vi "Configure Device.vi"(8 "error in":errorcluster, 11 "Vaisala Probe in":refnum<class "Vaisala.lvclass">) -> (0 "error out":errorcluster, 3 "Vaisala Probe out":refnum<class "Vaisala.lvclass">, 4 "SP":dbl, 5 "Settable?":bool)   [LabVIEW 2014, in "Vaisala Library.lvlib" / "Vaisala.lvclass"]
doc: "Configure the current instance of the Vaisala probe. In this case, we will get the correct address and then set the serial delayso that the probe responds in the correct amount of time. When configuration is done, make sure the session is closed."
uses:
  Vaisala.lvclass
  reusable/Session APIs/Serial/Serial Session.lvclass
  Configurable Device/Configurable Device.lvclass/Configurable Device.ctl
  reusable/Session APIs/File Access/Config Data/Config Data.lvclass/Config Data.ctl
  Vaisala.lvclass/Vaisala.ctl
  Configurable Device/Read ID.vi
  Configurable Device/Read Handle.vi
  Configurable Device/Read Log Session.vi
  Configurable Device/Accessors/Write type.vi
  Configurable Device/Accessors/Write controller_.vi
  reusable/Session APIs/File Access/Config Data/Accessors/Read Ref.vi
  Accessors/Write hSession.vi
  Accessors/Write Address.vi
  Configurable Device/Accessors/Write label.vi
  <vilib>/Utility/config.llb/Read Key (I32).vi
  <vilib>/Utility/config.llb/Read Key (String).vi
  Configurable Device/Configurable Device.lvclass
  reusable/Session APIs/File Access/Config Data/Config Data.lvclass
  <userlib>/_Session Fwk/Session - Root.lvclass
  <vilib>/Utility/config.llb/NI_LVConfig.lvlib
  reusable/Session APIs/Session Log/System Log.lvclass
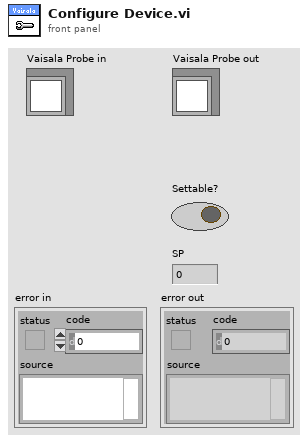
[diagram p1: front panel]
types:
  T1 = typedef "Config Data.lvclass/Config Session.ctl" = refnum<data-value>
  T2 = typedef "Session - Root.lvclass/Session Handle.ctl" = refnum<data-value>
  T3 = typedef "Serial Session.lvclass/Session Handle.ctl" = refnum<data-value>
  T4 = typedef "NI_LVConfig.lvlib/Config Data RefNum.ctl" = refnum<k1>
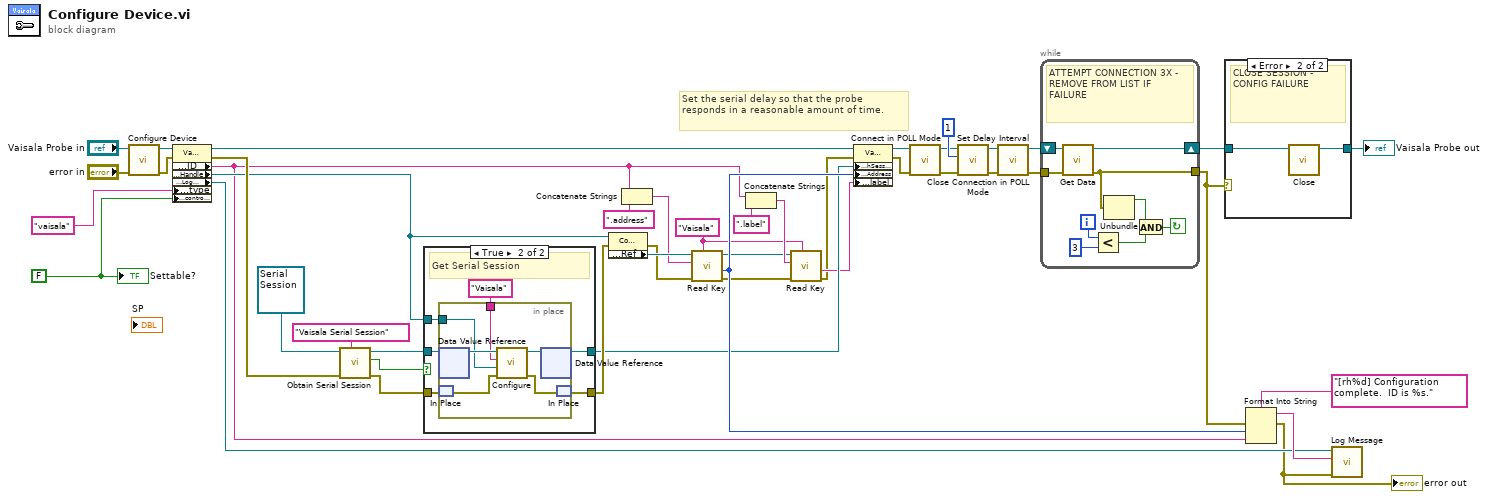
[diagram p0: block diagram]
diagram:
  w14 = FALSE ("controller_")
  w6 = "Vaisala" ("section")
  # "Set the serial delay so that the probe responds in a reasonable amount of time."
  n1 = call-parent "Configure Device.vi"("error in"="error in", "Device in"="Vaisala Probe in") -> ("error out"=w10:errorcluster, "Device out"=w11:refnum<class "Vaisala.lvclass">)  [unwired: 6 in, 2 out]
  n2 = property class="Vaisala"(reference=w11, error in=w10, "Accessors:type"="vaisala" ("type"), "Accessors:controller_"=w14) -> (reference out=w38:refnum<class "Vaisala.lvclass">, error out=w34:errorcluster, "Accessors:ID"=w1:string, "Accessors:Handle"=w31:T1, "Accessors:Log Session"=w32:T2)
  n3 = call "Obtain Serial Session.vi"("Session Name ()"="Vaisala Serial Session", "error in"=w34, "Serial Session in"=refnum<class "Serial Session.lvclass"> refnum) -> ("error out"=w35:errorcluster, "created new?"=w36:bool, "hSerial"=w39:T3)  [unwired: 6 in]
  n4 = case shown="True" w36 {
    tunnel: w39 -> [w47 w53]
    tunnel: w35 -> [w46 w50]
    tunnel: [w47 w52] -> w29
    tunnel: [w46 w49] -> w33
    tunnel: w31 -> [_ w51]
    frame False {
    }
    frame True {
      # "Get Serial Session"
      n5 = in-place {
        in-place-border: w51 -> [w54]
        in-place-border: "Vaisala" ("section") -> [w55]
        n6 = in-place-dvr #1(w53) -> (w59:refnum<class "Serial Session.lvclass">)  [unwired: 1 out]
        n7 = in-place-match #2(w50) -> (w58:errorcluster)
        n8 = call "Configure.vi"("error in"=w58, "Config Handle"=w54, "section"=w55, "Serial Session in"=w59) -> ("error out"=w57:errorcluster, "Serial Session out"=w56:refnum<class "Serial Session.lvclass">)  [unwired: 6 in]
        n9 = in-place-dvr #1(w56) -> (w52:T3)  [unwired: 1 out]
        n10 = in-place-match #2(w57) -> (w49:errorcluster)
      }
    }
  }
  n11 = property class="Config Data"(reference=w31, error in=w33) -> (error out=w30:errorcluster, "Accessors:Ref"=w45:T4)  [unwired: 1 out]
  n12 = Concatenate Strings(w1, ".address" ("string")) -> (w7:string)
  n13 = call-poly <vilib>:"Read Key.vi"("section"=w6, "error in (no error)"=w30, "key"=w7, "refnum"=w45) -> ("error out"=w3:errorcluster, "value"=w37:i32, "refnum out"=w5:T4)  [unwired: 4 in, 1 out]
  n14 = Concatenate Strings(w1, ".label" ("string")) -> (w8:string)
  n15 = call-poly <vilib>:"Read Key.vi"("section"=w6, "error in (no error)"=w3, "key"=w8, "refnum"=w5) -> ("error out"=w2:errorcluster, "value"=w4:string)  [unwired: 4 in, 2 out]
  n16 = property class="Vaisala"(reference=w38, error in=w2, "Accessors:hSession"=w29, "Accessors:Address"=w37, "Accessors:label"=w4) -> (reference out=w22:refnum<class "Vaisala.lvclass">, error out=w23:errorcluster)
  n17 = call "Connect in POLL Mode.vi"("error in"=w23, "Vaisala in"=w22) -> ("error out"=w26:errorcluster, "Vaisala out"=w27:refnum<class "Vaisala.lvclass">)  [unwired: 8 in]
  n18 = call "Set Delay Interval.vi"("error in"=w26, "Delay In"=u8 1, "Vaisala in"=w27) -> ("error out"=w24:errorcluster, "Vaisala out"=w25:refnum<class "Vaisala.lvclass">)  [unwired: 7 in]
  n19 = call "Close Connection in POLL Mode.vi"("error in"=w24, "Vaisala in"=w25) -> ("error out"=w19:errorcluster, "Vaisala out"=w21:refnum<class "Vaisala.lvclass">)  [unwired: 8 in]
  n20 = while {
    shift-right: [w66] -> w18
    shift-left: w21 -> [w65]
    tunnel: [w61] -> w20
    tunnel: w19 -> [w60]
    i -> [w68]
    stop <- w62 continue-if-true
    # "ATTEMPT CONNECTION 3X - REMOVE FROM LIST IF FAILURE"
    n21 = call-dynamic "Get Data.vi"("error in"=w60, "Cfg Dev in"=w65) -> ("error out"=w61:errorcluster, "Cfg Dev out"=w66:refnum<class "Vaisala.lvclass">)  [unwired: 7 in, 1 out]
    n22 = Less?(x=w68, y=3) -> (x < y?=w63:bool)
    n23 = Unbundle(w61) -> ("status"=w64:bool)  [unwired: 2 out]
    n24 = And(x=w64, y=w63) -> (x .and. y?=w62:bool)
  }
  n25 = case shown="Error" w20 {
    tunnel: w18 -> [w69 w71]
    tunnel: [w69 w70] -> w17
    frame No Error {
    }
    frame Error {
      # "CLOSE SESSION - CONFIG FAILURE"
      n26 = call-dynamic "Close.vi"("Cfg Dev in"=w71) -> ("Cfg Dev out"=w70:refnum<class "Vaisala.lvclass">)  [unwired: 9 in, 1 out]
    }
  }
  "Vaisala Probe out" <- w17
  n27 = Format Into String(format string="[rh%d] Configuration complete.  ID is %s.", error in=w20, w37, w1) -> (resulting string=w42:string, error out=w16:errorcluster)  [unwired: 1 in]
  "error out" <- w16
  n28 = call "Log Message.vi"("error in"=w16, "MSG In"=w42, "session in"=w32) -> ()  [unwired: 7 in, 2 out]
  "Settable?" <- w14
